vi "MecaDrivePoseEst_UpdateWithTime.vi"(8 "MecanumWheelSpeeds":T1 {"RearRightSpeed" format="%19.3f"; "RearLeftSpeed" format="%19.3f"; "FrontRightSpeed" format="%19.3f"; "FrontLeftSpeed" format="%19.3f"}, 9 "GyroAngle":T4={"VALUE"=0.0, "COS"=1.0, "SIN"=0.0} {"SIN" format="%13.4f"; "COS" format="%13.4f"; "VALUE" format="%13.4f"}, 10 "CurrentTimeSeconds":dbl, 11 "in MecaDrivePoseEstimate":T5={"M_VisionContR"=[], "m_nominal_dT"=0.0, "m_PrevTime_Sec"=0.0, "m_GyroOffset"={"VALUE"=0.0, "COS"=1.0, "SIN"=0.0}, "m_PrevAngle"={"VALUE"=0.0, "COS"=1.0, "SIN"=0.0}, "m_Observer"={"m_P"=[], "m_xHat"=[], "States"=0, "Outputs"=0, "m_ContR"=[], "m_ContQ"=[], "m_SigmasF"=[], "m_dT_Sec"=0.0, "MERWE_SCALED_SIGMA_PTS"={"m_Wm"=[], "States"=0, "Alpha"=0.0, "m_Wc"=[], "Kappa"=0}, "meanFuncX"=refnum, "meanFuncY"=refnum, "residualFuncX"=refnum, "residualFuncY"=refnum, "addFuncX"=refnum, "addFuncXExtra"=variant, "residualFuncYExtra"=variant, "residualFuncXExtra"=variant, "MeanFuncYExtra"=variant, "MeanFuncXExtra"=variant, "Inputs"=0}, "m_kinematics"={"FrontLeft"={"X"=0.0, "Y"=0.0}, "FrontRight"={"X"=0.0, "Y"=0.0}, "RearLeft"={"X"=0.0, "Y"=0.0}, "RearRight"={"X"=0.0, "Y"=0.0}, "InverseKinematics"=[[0.0, 1.0, -1.0, 0.0], [0.0, 1.0, 1.0, 0.0], [0.0, 1.0, 1.0, 0.0], [0.0, 1.0, -1.0, 0.0]], "ForwardKinematics"=[[0.0, 1.0, -1.0, 0.0], [0.0, 1.0, 1.0, 0.0], [0.0, 1.0, 1.0, 0.0], [0.0, 1.0, -1.0, 0.0]], "PrevCoR"={"X"=0.0, "Y"=0.0}}, "Pose_Buffer"={"TimeStamps"=[], "Pose"=[], "Min_TimeStamp"=0.0, "Max_TimeStamp"=0.0, "ItemCount"=0, "MaxBufferTime"=0.0}} {"Pose_Buffer"."Pose"."ROTATION"."SIN" format="%13.4f"; "Pose_Buffer"."Pose"."ROTATION"."COS" format="%13.4f"; "Pose_Buffer"."Pose"."ROTATION"."VALUE" format="%13.4f"; "Pose_Buffer"."Pose"."TRANSLATION"."Y" format="%14.3f"; "Pose_Buffer"."Pose"."TRANSLATION"."X" format="%14.3f"; "m_kinematics"."PrevCoR"."Y" format="%14.3f"; "m_kinematics"."PrevCoR"."X" format="%14.3f"; "m_kinematics"."RearRight"."Y" format="%14.3f"; "m_kinematics"."RearRight"."X" format="%14.3f"; "m_kinematics"."RearLeft"."Y" format="%14.3f"; "m_kinematics"."RearLeft"."X" format="%14.3f"; "m_kinematics"."FrontRight"."Y" format="%14.3f"; "m_kinematics"."FrontRight"."X" format="%14.3f"; "m_kinematics"."FrontLeft"."Y" format="%14.3f"; "m_kinematics"."FrontLeft"."X" format="%14.3f"; "m_PrevAngle"."SIN" format="%13.4f"; "m_PrevAngle"."COS" format="%13.4f"; "m_PrevAngle"."VALUE" format="%13.4f"; "m_GyroOffset"."SIN" format="%13.4f"; "m_GyroOffset"."COS" format="%13.4f"; "m_GyroOffset"."VALUE" format="%13.4f"}) -> (0 "Error":bool, 2 "Estimated Pose":T2 {"ROTATION"."SIN" format="%13.4f"; "ROTATION"."COS" format="%13.4f"; "ROTATION"."VALUE" format="%13.4f"; "TRANSLATION"."Y" format="%14.3f"; "TRANSLATION"."X" format="%14.3f"}, 3 "Out MecaDrivePoseEstimate":T5={"M_VisionContR"=[], "m_nominal_dT"=0.0, "m_PrevTime_Sec"=0.0, "m_GyroOffset"={"VALUE"=0.0, "COS"=1.0, "SIN"=0.0}, "m_PrevAngle"={"VALUE"=0.0, "COS"=1.0, "SIN"=0.0}, "m_Observer"={"m_P"=[], "m_xHat"=[], "States"=0, "Outputs"=0, "m_ContR"=[], "m_ContQ"=[], "m_SigmasF"=[], "m_dT_Sec"=0.0, "MERWE_SCALED_SIGMA_PTS"={"m_Wm"=[], "States"=0, "Alpha"=0.0, "m_Wc"=[], "Kappa"=0}, "meanFuncX"=refnum, "meanFuncY"=refnum, "residualFuncX"=refnum, "residualFuncY"=refnum, "addFuncX"=refnum, "addFuncXExtra"=variant, "residualFuncYExtra"=variant, "residualFuncXExtra"=variant, "MeanFuncYExtra"=variant, "MeanFuncXExtra"=variant, "Inputs"=0}, "m_kinematics"={"FrontLeft"={"X"=0.0, "Y"=0.0}, "FrontRight"={"X"=0.0, "Y"=0.0}, "RearLeft"={"X"=0.0, "Y"=0.0}, "RearRight"={"X"=0.0, "Y"=0.0}, "InverseKinematics"=[[0.0, 1.0, -1.0, 0.0], [0.0, 1.0, 1.0, 0.0], [0.0, 1.0, 1.0, 0.0], [0.0, 1.0, -1.0, 0.0]], "ForwardKinematics"=[[0.0, 1.0, -1.0, 0.0], [0.0, 1.0, 1.0, 0.0], [0.0, 1.0, 1.0, 0.0], [0.0, 1.0, -1.0, 0.0]], "PrevCoR"={"X"=0.0, "Y"=0.0}}, "Pose_Buffer"={"TimeStamps"=[], "Pose"=[], "Min_TimeStamp"=0.0, "Max_TimeStamp"=0.0, "ItemCount"=0, "MaxBufferTime"=0.0}} {"Pose_Buffer"."Pose"."ROTATION"."SIN" format="%13.4f"; "Pose_Buffer"."Pose"."ROTATION"."COS" format="%13.4f"; "Pose_Buffer"."Pose"."ROTATION"."VALUE" format="%13.4f"; "Pose_Buffer"."Pose"."TRANSLATION"."Y" format="%14.3f"; "Pose_Buffer"."Pose"."TRANSLATION"."X" format="%14.3f"; "m_kinematics"."PrevCoR"."Y" format="%14.3f"; "m_kinematics"."PrevCoR"."X" format="%14.3f"; "m_kinematics"."RearRight"."Y" format="%14.3f"; "m_kinematics"."RearRight"."X" format="%14.3f"; "m_kinematics"."RearLeft"."Y" format="%14.3f"; "m_kinematics"."RearLeft"."X" format="%14.3f"; "m_kinematics"."FrontRight"."Y" format="%14.3f"; "m_kinematics"."FrontRight"."X" format="%14.3f"; "m_kinematics"."FrontLeft"."Y" format="%14.3f"; "m_kinematics"."FrontLeft"."X" format="%14.3f"; "m_PrevAngle"."SIN" format="%13.4f"; "m_PrevAngle"."COS" format="%13.4f"; "m_PrevAngle"."VALUE" format="%13.4f"; "m_GyroOffset"."SIN" format="%13.4f"; "m_GyroOffset"."COS" format="%13.4f"; "m_GyroOffset"."VALUE" format="%13.4f"})   [LabVIEW 2019, in "Trajectory_Library.lvlib"]
doc: "Updates the the Unscented Kalman Filter using only wheel encoder information. This should be called every loop, and the correct loop period must be passed into the constructor of this class.\n \nInputs:\n - SwervePoseEst -- Data cluster containing SwervePoseEst data\n - currentTimeSeconds Time at which this method was called, in seconds.\n - gyroAngle The current gyroscope angle.\n - moduleStates The current velocities and rotations of the swerve modules.\n\nOutputs:\n - outSwevePoseEst -- Updated data cluster \n - EstimatedPose -- The estimated pose of the robot in meters.\n - Error -- If TRUE, an error occured."
uses:
  Trajectory_Library.lvlib
  MECA_DRIVE_POSE_EST.ctl
  <vilib>/Analysis/Matrix/Datatypes/RealMatrix.ctl
  ROTATION2D.ctl
  UNSCENTED_KALMAN_FILTER.ctl
  MERWE_SCALED_SIGMA_PTS.ctl
  CALLBACK_FUNC_TYPE.ctl
  MECA_DRIVE_KINEMATICS.ctl
  TRANSLATION2D.ctl
  TIME_INTERPOLATABLE_POSE2D.ctl
  POSE2D.ctl
  MECA_WHEEL_SPEEDS.ctl
  Rotation2d_RotateBy.vi
  MatBuilder_Create.vi
  Rotation2d_UnaryMinus.vi
  TimeInterpPose2d_CleanUp.vi
  Rotation2d_CreateXY.vi
  Rotation2d_CreateAngle.vi
  Util_CalcDist.vi
  MecaDrivePoseEst_Kalman_F_Callback.vi
  MecaDrivePoseEst_Kalman_H_Callback.vi
  <vilib>/gmath/interp.llb/Search Ordered Table.vi
  <vilib>/Analysis/Matrix/NI_Matrix.lvlib
panel:
  # "<3, 3>"
  # "State Estimate <Statess,1>"
  # "<States, States>"
  # "<States, ?>"
  # "<Statess,  States>"
  # "<Outputs, Outputs>"
  # "<?, 1>"
  # "<?, 1>"
  # "<3, 3>"
  # "State Estimate <Statess,1>"
  # "<States, States>"
  # "<States, ?>"
  # "<Statess,  States>"
  # "<Outputs, Outputs>"
  # "<?, 1>"
  # "<?, 1>"
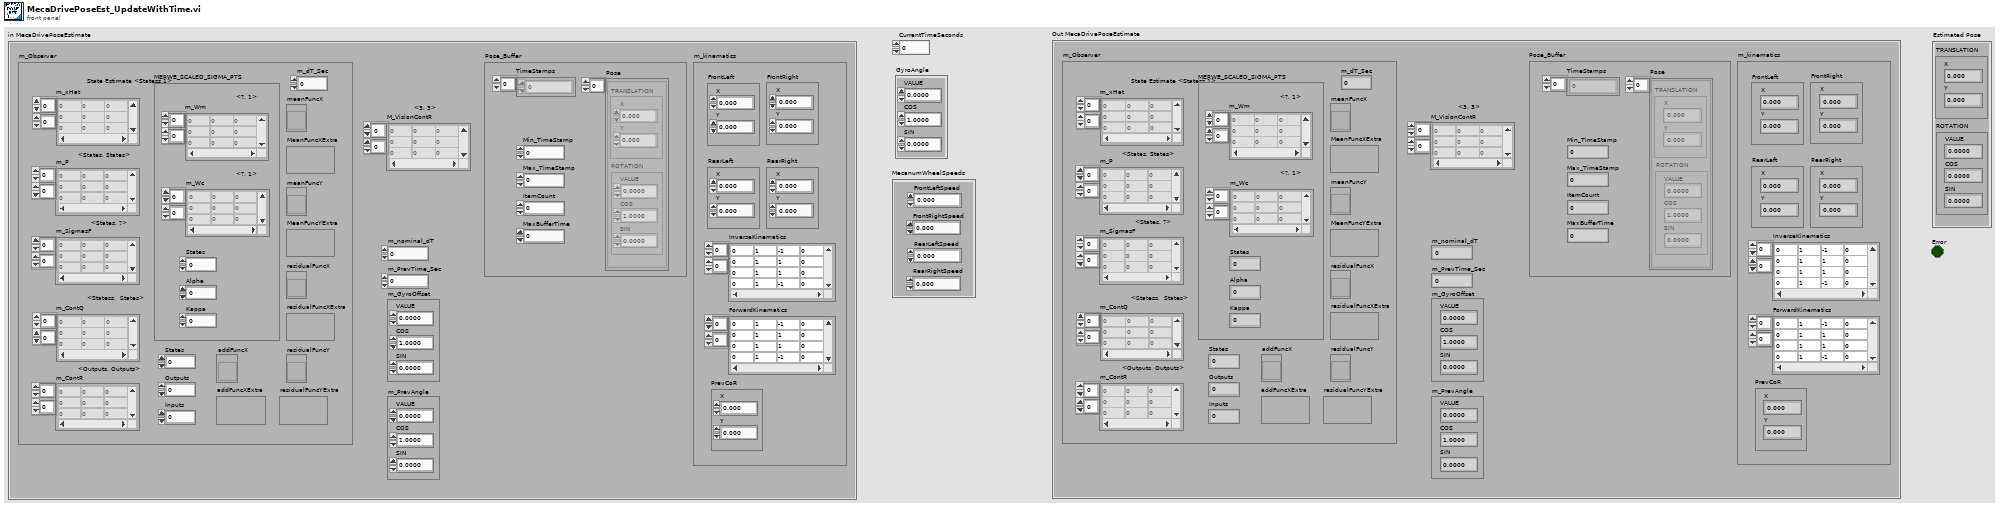
[diagram p1: front panel]
types:
  T1 = typedef "Trajectory_Library.lvlib/MECA_WHEEL_SPEEDS.ctl" = cluster{"FrontLeftSpeed":dbl, "FrontRightSpeed":dbl, "RearLeftSpeed":dbl, "RearRightSpeed":dbl}
  T2 = typedef "Trajectory_Library.lvlib/POSE2D.ctl" = cluster{"TRANSLATION":T3, "ROTATION":T4}
  T3 = typedef "Trajectory_Library.lvlib/TRANSLATION2D.ctl" = cluster{"X":dbl, "Y":dbl}
  T4 = typedef "Trajectory_Library.lvlib/ROTATION2D.ctl" = cluster{"VALUE":dbl, "COS":dbl, "SIN":dbl}
  T5 = typedef "Trajectory_Library.lvlib/MECA_DRIVE_POSE_EST.ctl" = cluster{"M_VisionContR":T6, "m_nominal_dT":dbl, "m_PrevTime_Sec":dbl, "m_GyroOffset":T4, "m_PrevAngle":T4, "m_Observer":T7, "m_kinematics":T10, "Pose_Buffer":T11}
  T6 = typedef "NI_Matrix.lvlib/RealMatrix.ctl" = dbl[][]
  T7 = typedef "Trajectory_Library.lvlib/UNSCENTED_KALMAN_FILTER.ctl" = cluster{"m_P":T6, "m_xHat":T6, "States":i32, "Outputs":i32, "m_ContR":T6, "m_ContQ":T6, "m_SigmasF":T6, "m_dT_Sec":dbl, "MERWE_SCALED_SIGMA_PTS":T8, "meanFuncX":T9, "meanFuncY":T9, "residualFuncX":T9, "residualFuncY":T9, "addFuncX":T9, "addFuncXExtra":variant, "residualFuncYExtra":variant, "residualFuncXExtra":variant, "MeanFuncYExtra":variant, "MeanFuncXExtra":variant, "Inputs":i32}
  T8 = typedef "Trajectory_Library.lvlib/MERWE_SCALED_SIGMA_PTS.ctl" = cluster{"m_Wm":T6, "States":i32, "Alpha":dbl, "m_Wc":T6, "Kappa":i32}
  T9 = typedef "Trajectory_Library.lvlib/CALLBACK_FUNC_TYPE.ctl" = refnum<vi>
  T10 = typedef "Trajectory_Library.lvlib/MECA_DRIVE_KINEMATICS.ctl" = cluster{"FrontLeft":T3, "FrontRight":T3, "RearLeft":T3, "RearRight":T3, "InverseKinematics":T6, "ForwardKinematics":T6, "PrevCoR":T3}
  T11 = typedef "Trajectory_Library.lvlib/TIME_INTERPOLATABLE_POSE2D.ctl" = cluster{"TimeStamps":dbl[], "Pose":T2[], "Min_TimeStamp":dbl, "Max_TimeStamp":dbl, "ItemCount":i32, "MaxBufferTime":dbl}
  T12 = typedef "Trajectory_Library.lvlib/CHASSIS_SPEEDS.ctl" = cluster{"vX":dbl, "vY":dbl, "vOmega":dbl}
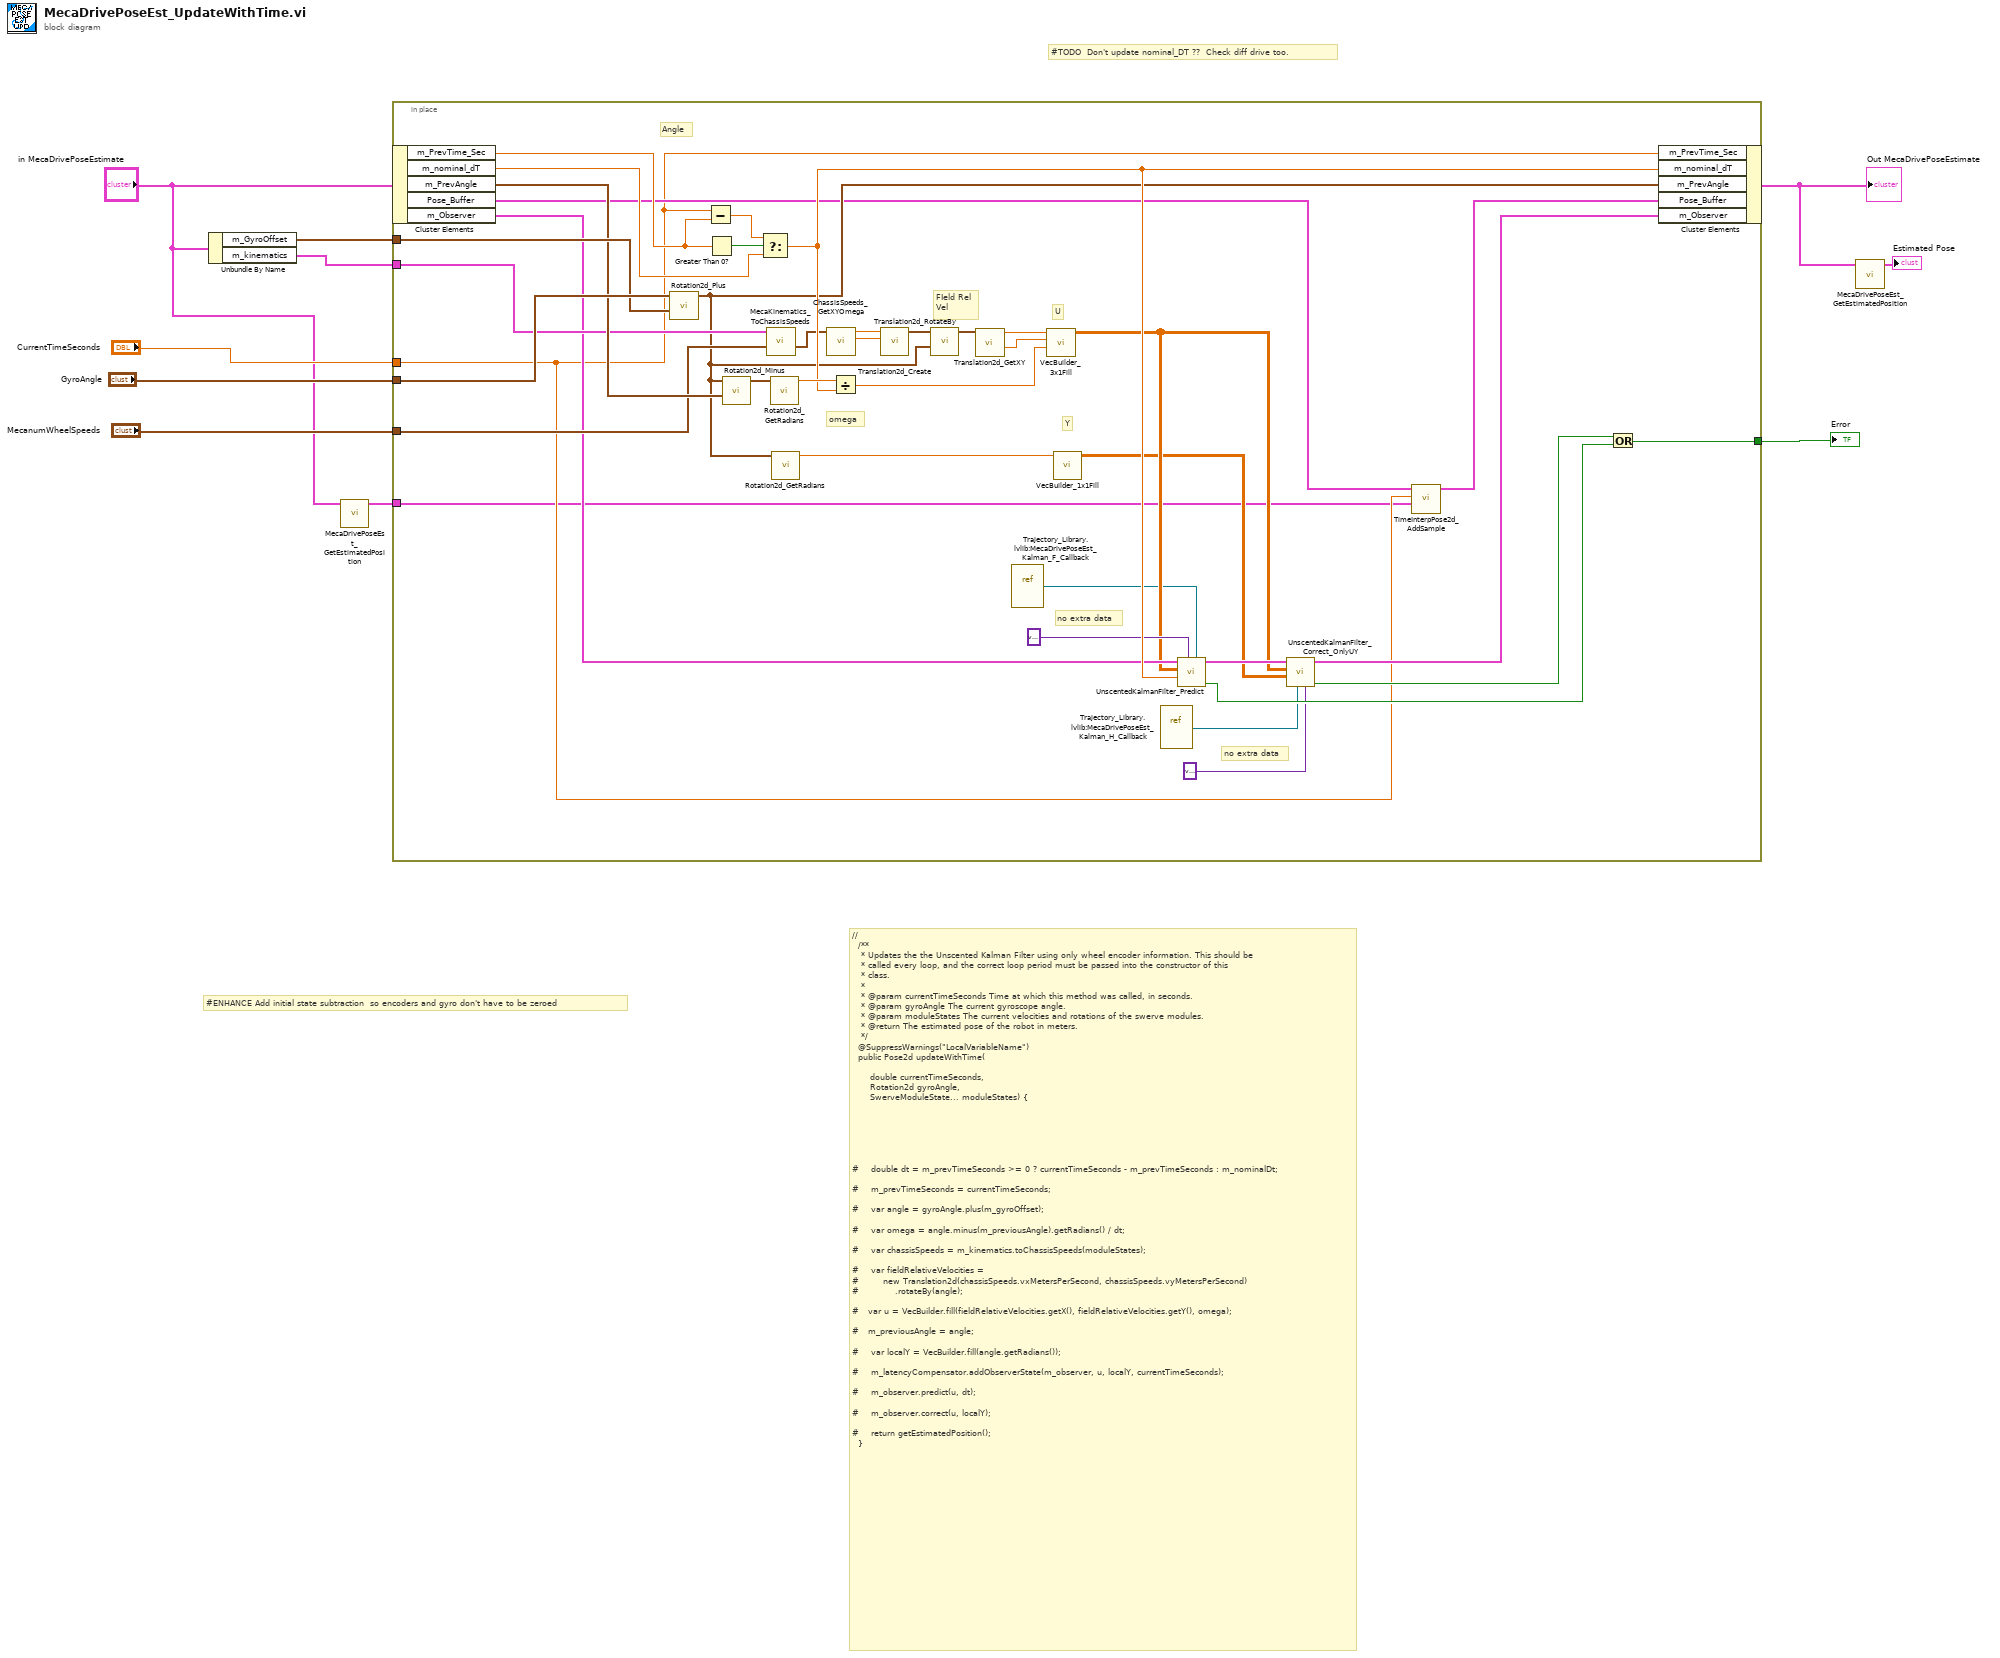
[diagram p0: block diagram]
diagram:
  # "#TODO  Don't update nominal_DT ??  Check diff drive too."
  # "#ENHANCE Add initial state subtraction  so encoders and gyro don't have to be zeroed"
  # "//\n  /**\n   * Updates the the Unscented Kalman Filter using only wheel encoder information. This should be\n   * called every loop, and the correct loop period must be passed into the constructor of this\n   * class.\n   *\n   * @param currentTimeSeconds Time at which this method was called, in seconds.\n   * @param gyroAngle The current gyroscope angle.\n   * @param moduleStates The current velocities and rotations of the swerve modules.\n   * @return The estimated pose of the robot in meters.\n   */\n  @SuppressWarnings(\"LocalVariableName\")\n  public Pose2d updateWithTime(\n\n      double currentTimeSeconds, \n      Rotation2d gyroAngle, \n      SwerveModuleState... moduleStates) {\n\n\n\n\n\n\n#    double dt = m_prevTimeSeconds >= 0 ? currentTimeSeconds - m_prevTimeSeconds : m_nominalDt;\n\n#    m_prevTimeSeconds = currentTimeSeconds;\n\n#    var angle = gyroAngle.plus(m_gyroOffset);\n\n#    var omega = angle.minus(m_previousAngle).getRadians() / dt;\n\n#    var chassisSpeeds = m_kinematics.toChassisSpeeds(moduleStates);\n\n#    var fieldRelativeVelocities =\n#        new Translation2d(chassisSpeeds.vxMetersPerSecond, chassisSpeeds.vyMetersPerSecond)\n#            .rotateBy(angle);\n\n#   var u = VecBuilder.fill(fieldRelativeVelocities.getX(), fieldRelativeVelocities.getY(), omega);\n \n#   m_previousAngle = angle;\n\n#    var localY = VecBuilder.fill(angle.getRadians());\n\n#    m_latencyCompensator.addObserverState(m_observer, u, localY, currentTimeSeconds);\n\n#    m_observer.predict(u, dt);\n\n#    m_observer.correct(u, localY);\n\n#    return getEstimatedPosition();\n  }"
  n1 = Unbundle By Name("in MecaDrivePoseEstimate") -> ("m_GyroOffset"=w8:T4, "m_kinematics"=w4:T10)
  n2 = call "MecaDrivePoseEst_GetEstimatedPosition.vi"("in PoseDrivePoseEstimate"="in MecaDrivePoseEstimate") -> ("Estimated Pose"=w1:T2)  [unwired: 10 in]
  n3 = in-place {
    in-place-border: "CurrentTimeSeconds" -> [w14]
    in-place-border: "GyroAngle" -> [w45]
    in-place-border: w8 -> [w44]
    in-place-border: [w37] -> w5
    in-place-border: w4 -> [w31]
    in-place-border: "MecanumWheelSpeeds" -> [w30]
    in-place-border: w1 -> [w13]
    # "FIeld Rel\nVel"
    # "omega"
    # "Angle"
    # "no extra data"
    # "no extra data"
    # "Y"
    # "U"
    n4 = in-place-cluster #1("in MecaDrivePoseEstimate") -> ("m_PrevTime_Sec"=w47:dbl, "m_nominal_dT"=w42:dbl, "m_PrevAngle"=w32:T4, "Pose_Buffer"=w16:T11, "m_Observer"=w19:T7)
    n5 = call "Rotation2d_Plus.vi"("other ROTATION"=w44, "in ROTATION"=w45) -> ("out ROTATION"=w25:T4)  [unwired: 9 in]
    n6 = Subtract(x=w14, y=w47) -> (x-y=w46:dbl)
    n7 = Greater Than 0?(x=w47) -> (x > 0?=w48:bool)
    n8 = call "Rotation2d_Minus.vi"("other ROTATION"=w32, "in ROTATION"=w25) -> ("out ROTATION"=w43:T4)  [unwired: 9 in]
    n9 = Select(t=w46, s=w48, f=w42) -> (s? t:f=w36:dbl)
    n10 = call "MecaKinematics_ToChassisSpeeds.vi"("MECA_WHEEL_SPEEDS"=w30, "in MECA_DRIVE_KINEMATICS"=w31) -> ("ChassisSpeeds"=w29:T12)  [unwired: 9 in]
    n11 = call "Rotation2d_GetRadians.vi"("in ROTATION"=w43) -> ("AngleRadians"=w41:dbl)  [unwired: 10 in]
    n12 = call "Rotation2d_GetRadians.vi"("in ROTATION"=w25) -> ("AngleRadians"=w20:dbl)  [unwired: 10 in]
    n13 = call "ChassisSpeeds_GetXYOmega.vi"("CHASSIS"=w29) -> ("vY"=w27:dbl, "vX"=w28:dbl)  [unwired: 8 in, 1 out]
    n14 = Divide(x=w41, y=w36) -> (x/y=w21:dbl)
    n15 = call "Translation2d_Create.vi"("Y"=w27, "X"=w28) -> ("TRANSLATION"=w26:T3)  [unwired: 9 in]
    n16 = call "Translation2d_RotateBy.vi"("other Rotation"=w25, "In Translation"=w26) -> ("Out Translation"=w24:T3)  [unwired: 9 in]
    n17 = call "Translation2d_GetXY.vi"("In Translation"=w24) -> ("Y"=w22:dbl, "X"=w23:dbl)  [unwired: 9 in]
    n18 = vi-ref "Trajectory_Library.lvlib:MecaDrivePoseEst_Kalman_F_Callback.vi"() -> (w12:refnum<vi>)
    n19 = call "VecBuilder_3x1Fill.vi"("R2"=w21, "R1"=w22, "R0"=w23) -> ("output matrix"=w18:T6)  [unwired: 8 in]
    n20 = call "VecBuilder_1x1Fill.vi"("R0_C0"=w20) -> ("output matrix"=w17:T6)  [unwired: 10 in]
    n21 = vi-ref "Trajectory_Library.lvlib:MecaDrivePoseEst_Kalman_H_Callback.vi"() -> (w11:refnum<vi>)
    n22 = call "UnscentedKalmanFilter_Predict.vi"("f_Func"=w12, "F_Func_ExtraData"=variant, "dT_Seconds"=w36, "U"=w18, "in UnscentedKalmanFiilter"=w19) -> ("Error"=w38:bool, "out UnscentedKalmanFiilter"=w40:T7)  [unwired: 5 in]
    n23 = call "UnscentedKalmanFilter_Correct_OnlyUY.vi"("H_ExtraData"=variant ("F_Func_ExtraData"), "H_Func"=w11, "Y"=w17, "U"=w18, "in UnscentedKalmanFiilter"=w40) -> ("Error"=w39:bool, "out UnscentedKalmanFiilter"=w33:T7)  [unwired: 5 in]
    n24 = call "TimeInterpPose2d_AddSample.vi"("Pose"=w13, "TimeStamp"=w14, "in TimeInterpPose"=w16) -> ("out TimeInterpPose"=w15:T11)  [unwired: 7 in, 1 out]
    n25 = Or(x=w39, y=w38) -> (x .or. y?=w37:bool)
    n26 = in-place-cluster #1("m_PrevTime_Sec"=w14, "m_nominal_dT"=w36, "m_PrevAngle"=w25, "Pose_Buffer"=w15, "m_Observer"=w33) -> (w7:T5)
  }
  "Out MecaDrivePoseEstimate" <- w7
  "Error" <- w5
  n27 = call "MecaDrivePoseEst_GetEstimatedPosition.vi"("in PoseDrivePoseEstimate"=w7) -> ("Estimated Pose"=→"Estimated Pose":T2)  [unwired: 10 in]
